vi "MeasureStateStub.vi"() -> ()   [LabVIEW 2013]
panel:
  in  "State":cluster{bool, "CalibrationState":u32}
  # "CalibrationDone"
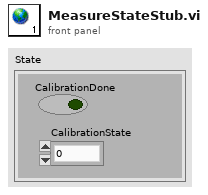
[diagram p1: front panel]
diagram:
